vi "Parse CSV File.vi"(11 "String":string) -> (3 "Array":string[][](array[string]))   [LabVIEW 2025, in "Project.lvclass"]
doc: "Convert CSV string to 2D Array."
uses:
  Project.lvclass
  Project.lvclass/Project.ctl
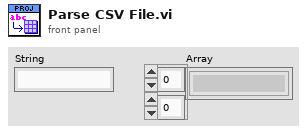
[diagram p1: front panel]
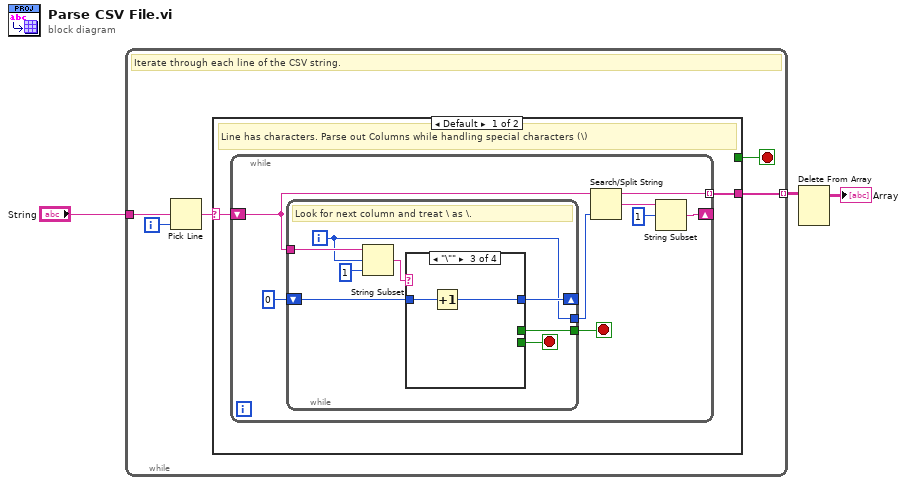
[diagram p0: block diagram]
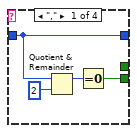
[diagram p2: hidden frame]
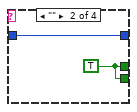
[diagram p3: hidden frame]
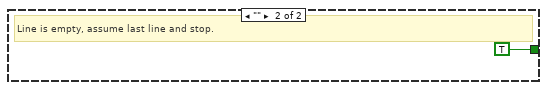
[diagram p5: hidden frame]
diagram:
  n1 = while {
    tunnel: "String" -> [w7]
    tunnel: [w4] -> w1 mode=indexing
    i -> [w8]
    stop <- w5 stop-if-true
    # "Iterate through each line of the CSV string."
    n2 = Pick Line(multi-line string=w7, line index=w8) -> (output string=w6:string)  [unwired: 1 in]
    n3 = case shown="Default" w6 {
      selector: w6 -> [w10 _]
      tunnel: [_ TRUE] -> w5
      tunnel: [w9 _] -> w4
      frame Default {
        # "Line has characters. Parse out Columns while handling special characters (\\)"
        n4 = while {
          tunnel: [w15] -> w9 mode=indexing
          shift-right: [w11] -> _
          shift-left: w10 -> [w17]
          stop <- w16 stop-if-true
          n5 = while {
            tunnel: w17 -> [w21]
            shift-right: [w23] -> _
            shift-left: 0 -> [w24]
            tunnel: [w20] -> w16
            tunnel: [w19] -> w14
            i -> [w19]
            stop <- w22 stop-if-true
            # "Look for next column and treat \\ as \\."
            n6 = String Subset(string=w21, offset (0)=w19, length (rest)=1 ("length (rest)")) -> (substring=w25:string)
            n7 = case shown="\"\\\"\"" w25 {
              tunnel: w24 -> [w30 w31 w34 w35]
              tunnel: [w30 w31 w33 w35] -> w23
              tunnel: [w27 w32 _ _] -> w22
              tunnel: [_ w32 _ _] -> w20
              frame "," {
                n8 = Quotient & Remainder(x=w30, y=2) -> (x-y*floor(x/y)=w28:i32)  [unwired: 1 out]
                n9 = Equal To 0?(x=w28) -> (x = 0?=w27:bool)
              }
              frame "" {
                w32 = TRUE
              }
              frame "\"" {
                n10 = Increment(x=w34) -> (x+1=w33:i32)
              }
              frame Default {
              }
            }
          }
          n11 = Search/Split String(string=w17, offset (0)=w14) -> (substring before match=w15:string, match + rest of string=w13:string)  [unwired: 1 in, 1 out]
          n12 = String Subset(string=w13, offset (0)=1) -> (substring=w11:string)  [unwired: 1 in]
        }
      }
      frame "" {
        # "Line is empty, assume last line and stop."
      }
    }
  }
  n13 = Delete From Array(array=w1) -> (array with subset deleted=→"Array":string[][])  [unwired: 3 in, 1 out]
